vi "Duplicate Name Error Test.vi"() -> (0 "error out":errorcluster, 1 "Success Error on Replace Line":bool, 2 "Success Error on Write Lines":bool, 3 "Success Error on Add":bool)   [LabVIEW 2014, in "DAQmx Module Tests.lvlib"]
doc: "Tests the Add Line and Remove Line functions."
uses:
  DAQmx Module Tests.lvlib
  module/configuration/Line.ctl
  <vilib>/NI/Tag Bus Module Framework/channel/TBM channel.lvclass
  module/configuration/Measurement Type.ctl
  module/configuration/Parameters.ctl
  module/configuration/Get Line Name.vi
  <vilib>/NI/Tag Bus Module Framework/module configuration/FindDuplicate.vi
  <vilib>/Utility/error.llb/Error Cluster From Error Code.vi
  module/configuration/DAQmx Module Configuration.lvclass
  editor node/DAQmx Module Editor Node.lvclass
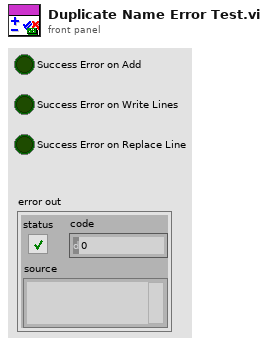
[diagram p1: front panel]
types:
  T1 = typedef "DAQmx Module Configuration.lvclass/Measurement Type.ctl" = enum16{"Digital Input", "Digital Output", "Voltage Input", "Voltage Output", "Current Input", "Current Output", "RTD", "Thermocouple", "Strain"}
  T2 = typedef "Daqmx Module configuration.lvclass/Line.ctl" = cluster{"channel":refnum<class "TBM channel.lvclass">, "Physical Channel":string, "Measurement Type":T3, "Parameters":T4}
  T3 = typedef "Daqmx Module configuration.lvclass/Measurement Type.ctl" = enum16{"Digital Input", "Digital Output", "Voltage Input", "Voltage Output", "Current Input", "Current Output", "RTD", "Thermocouple", "Strain"}
  T4 = typedef "Daqmx Module configuration.lvclass/Parameters.ctl" = cluster{"Digital Config":cluster{"Invert Lines?":bool}, "Voltage Config":cluster{"Maximum Value (V)":dbl, "Minimum Value (V)":dbl, "in terminal configuration (V)":i32, "out terminal configuration (V)":i32}, "Current Config":cluster{"Maximum Value (A)":dbl, "Minimum Value (A)":dbl, "shunt resistor location":i32, "input terminal configuration (C)":i32, "external shunt resistor value":dbl}, "RTD Config":cluster{"Maximum Value (°C)":dbl, "Minimum Value (°C)":dbl, "resistance configuration":i32, "r0":dbl, "current excitation value":dbl, "rtd type":i32, "current excitation source":i32}, "Thermocouple Config":cluster{"Minimum Value (C)":dbl, "Maximum Value (C)":dbl, "thermocouple type":i32, "cjc source":i32, "cjc value":dbl}, "Strain Config":cluster{"Maximum Value":dbl, "Minimum Value":dbl, "bridge information":cluster{"strain configuration":i32, "lead wire resistance":dbl, "initial bridge voltage":dbl, "voltage excitation source":i32, "voltage excitation value":dbl}, "strain gage information":cluster{"gage factor":dbl, "nominal gage resistance":dbl, "poisson ratio":dbl}}}
  T5 = typedef "TBM channel.lvclass/channel classification.ctl" = enum16{"input data", "output data", "processing parameter", "processing result"}
  T6 = typedef "tag bus.lvlib/tag descriptor.lvclass/Data Type.ctl" = enum16{"Double", "Single", "I64", "I32", "I16", "I8", "U64", "U32", "U16", "U8", "Boolean", "String", "Array of Double", "Array of Single", "Array of I64", "Array of I32", "Array of I16", "Array of I8", "Array of U64", "Array of U32", "Array of U16", "Array of U8", "Array of Boolean", "Array of String"}
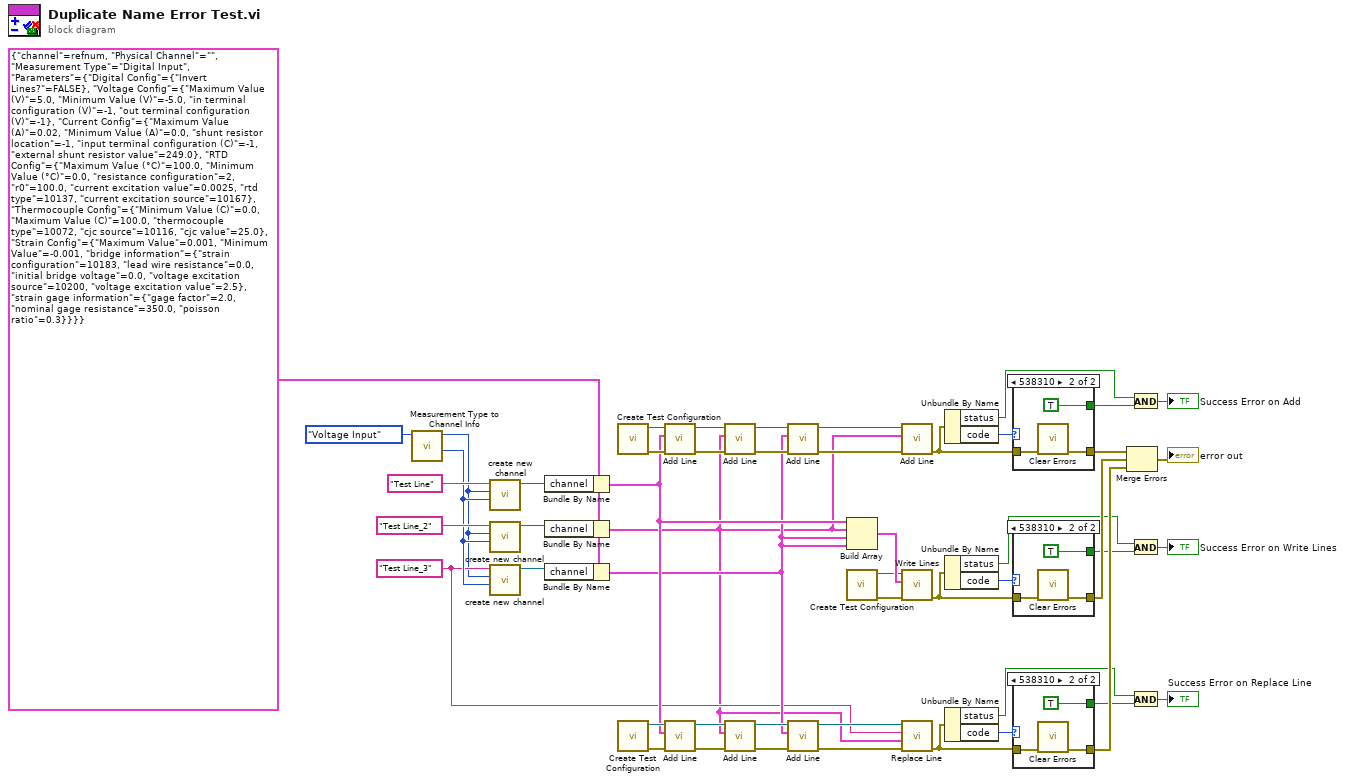
[diagram p0: block diagram]
diagram:
  w18 = "Test Line_3" ("channel name")
  w44 = T2 {"channel"=refnum, "Physical Channel"="", "Measurement Type"=enum."Digital Input", "Parameters"={"Digital Config"={"Invert Lines?"=FALSE}, "Voltage Config"={"Maximum Value (V)"=5.0, "Minimum Value (V)"=-5.0, "in terminal configuration (V)"=-1, "out terminal configuration (V)"=-1}, "Current Config"={"Maximum Value (A)"=0.02, "Minimum Value (A)"=0.0, "shunt resistor location"=-1, "input terminal configuration (C)"=-1, "external shunt resistor value"=249.0}, "RTD Config"={"Maximum Value (°C)"=100.0, "Minimum Value (°C)"=0.0, "resistance configuration"=2, "r0"=100.0, "current excitation value"=0.0025, "rtd type"=10137, "current excitation source"=10167}, "Thermocouple Config"={"Minimum Value (C)"=0.0, "Maximum Value (C)"=100.0, "thermocouple type"=10072, "cjc source"=10116, "cjc value"=25.0}, "Strain Config"={"Maximum Value"=0.001, "Minimum Value"=-0.001, "bridge information"={"strain configuration"=10183, "lead wire resistance"=0.0, "initial bridge voltage"=0.0, "voltage excitation source"=10200, "voltage excitation value"=2.5}, "strain gage information"={"gage factor"=2.0, "nominal gage resistance"=350.0, "poisson ratio"=0.3}}}} ("Line")
  n1 = call "Measurement Type to Channel Info.vi"("Measurement Type"=Measurement_Type."Voltage Input") -> ("channel classification"=w39:T5, "Data Type"=w2:T6)  [unwired: 8 in]
  n2 = call <vilib>:"create new channel.vi"("channel classification"=w39, "data type"=w2, "channel name"="Test Line") -> ("channel"=w50:refnum<class "TBM channel.lvclass">)  [unwired: 8 in]
  n3 = call <vilib>:"create new channel.vi"("channel classification"=w39, "data type"=w2, "channel name"="Test Line_2") -> ("channel"=w46:refnum<class "TBM channel.lvclass">)  [unwired: 8 in]
  n4 = call <vilib>:"create new channel.vi"("channel classification"=w39, "data type"=w2, "channel name"=w18) -> ("channel"=w45:refnum<class "TBM channel.lvclass">)  [unwired: 8 in]
  n5 = Bundle By Name(cluster=w44, "channel"=w50) -> (w21:T2)
  n6 = Bundle By Name(cluster=w44, "channel"=w46) -> (w17:T2)
  n7 = Bundle By Name(cluster=w44, "channel"=w45) -> (w20:T2)
  n8 = call "Create Test Configuration.vi"() -> ("error out"=w49:errorcluster, "Module Configuration"=w51:refnum<class "DAQmx Module Configuration.lvclass">)  [unwired: 6 in, 4 out]
  n9 = call "Create Test Configuration.vi"() -> ("error out"=w23:errorcluster, "Module Configuration"=w22:refnum<class "DAQmx Module Configuration.lvclass">)  [unwired: 6 in, 4 out]
  n10 = call "Add Line.vi"("error in"=w49, "Line"=w21, "Daqmx Module configuration in"=w51) -> ("error out"=w43:errorcluster, "Daqmx Module configuration out"=w40:refnum<class "DAQmx Module Configuration.lvclass">)  [unwired: 6 in, 1 out]
  n11 = call "Add Line.vi"("error in"=w23, "Line"=w21, "Daqmx Module configuration in"=w22) -> ("error out"=w24:errorcluster, "Daqmx Module configuration out"=w27:refnum<class "DAQmx Module Configuration.lvclass">)  [unwired: 6 in, 1 out]
  n12 = call "Add Line.vi"("error in"=w43, "Line"=w17, "Daqmx Module configuration in"=w40) -> ("error out"=w42:errorcluster, "Daqmx Module configuration out"=w41:refnum<class "DAQmx Module Configuration.lvclass">)  [unwired: 6 in, 1 out]
  n13 = call "Add Line.vi"("error in"=w24, "Line"=w17, "Daqmx Module configuration in"=w27) -> ("error out"=w25:errorcluster, "Daqmx Module configuration out"=w26:refnum<class "DAQmx Module Configuration.lvclass">)  [unwired: 6 in, 1 out]
  n14 = call "Add Line.vi"("error in"=w42, "Line"=w20, "Daqmx Module configuration in"=w41) -> ("error out"=w37:errorcluster, "Daqmx Module configuration out"=w38:refnum<class "DAQmx Module Configuration.lvclass">)  [unwired: 6 in, 1 out]
  n15 = call "Add Line.vi"("error in"=w25, "Line"=w20, "Daqmx Module configuration in"=w26) -> ("error out"=w16:errorcluster, "Daqmx Module configuration out"=w19:refnum<class "DAQmx Module Configuration.lvclass">)  [unwired: 6 in, 1 out]
  n16 = Build Array(w21, w17, w20, w20) -> (w34:T2[])
  n17 = call "Create Test Configuration.vi"() -> ("error out"=w15:errorcluster, "Module Configuration"=w33:refnum<class "DAQmx Module Configuration.lvclass">)  [unwired: 6 in, 4 out]
  n18 = call "Add Line.vi"("error in"=w37, "Line"=w17, "Daqmx Module configuration in"=w38) -> ("error out"=w35:errorcluster)  [unwired: 6 in, 2 out]
  n19 = call "Write Lines.vi"("error in (no error)"=w15, "Lines"=w34, "Daqmx Module configuration in"=w33) -> ("error out"=w31:errorcluster)  [unwired: 7 in, 1 out]
  n20 = call "Replace Line.vi"("error in"=w16, "New Line"=w17, "Line Name"=w18, "Daqmx Module configuration in"=w19) -> ("error out"=w13:errorcluster)  [unwired: 5 in, 2 out]
  n21 = Unbundle By Name(w35) -> ("status"=w10:bool, "code"=w36:i32)
  n22 = Unbundle By Name(w31) -> ("status"=w5:bool, "code"=w32:i32)
  n23 = Unbundle By Name(w13) -> ("status"=w6:bool, "code"=w14:i32)
  n24 = case shown="538310" w36 {
    tunnel: w35 -> [w52 w55]
    tunnel: [w52 w54] -> w30
    tunnel: [_ TRUE ("Success Error on Add")] -> w11
    frame 0, Default {
    }
    frame 538310 {
      n25 = call <vilib>:"Clear Errors.vi"("error in (no error)"=w55) -> ("error out"=w54:errorcluster)  [unwired: 5 in, 1 out]
    }
  }
  n26 = case shown="538310" w32 {
    tunnel: w31 -> [w56 w59]
    tunnel: [w56 w58] -> w29
    tunnel: [_ TRUE ("Success Error on Add")] -> w4
    frame 0, Default {
    }
    frame 538310 {
      n27 = call <vilib>:"Clear Errors.vi"("error in (no error)"=w59) -> ("error out"=w58:errorcluster)  [unwired: 5 in, 1 out]
    }
  }
  n28 = case shown="538310" w14 {
    tunnel: w13 -> [w60 w63]
    tunnel: [w60 w62] -> w12
    tunnel: [_ TRUE ("Success Error on Add")] -> w7
    frame 0, Default {
    }
    frame 538310 {
      n29 = call <vilib>:"Clear Errors.vi"("error in (no error)"=w63) -> ("error out"=w62:errorcluster)  [unwired: 5 in, 1 out]
    }
  }
  n30 = Merge Errors(w30, w29, w12) -> (→"error out":errorcluster)
  n31 = And(x=w10, y=w11) -> (x .and. y?=→"Success Error on Add":bool)
  n32 = And(x=w5, y=w4) -> (x .and. y?=→"Success Error on Write Lines":bool)
  n33 = And(x=w6, y=w7) -> (x .and. y?=→"Success Error on Replace Line":bool)
